vi "Read IP.vi"(8 "error in (no error)":errorcluster, 11 "RSeries_CAM in":refnum<class "RSeries_CAM.lvclass">) -> (0 "error out":errorcluster, 2 "IP":string, 3 "RSeries_CAM out":refnum<class "RSeries_CAM.lvclass">)   [LabVIEW 2024, in "RSeries_CAM.lvlib" / "RSeries_CAM.lvclass"]
uses:
  RSeries_CAM.lvclass
  RSeries_CAM.lvclass/RSeries_CAM.ctl
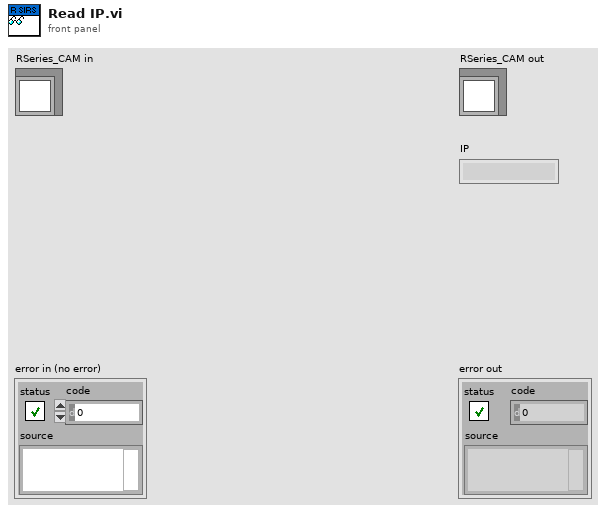
[diagram p1: front panel]
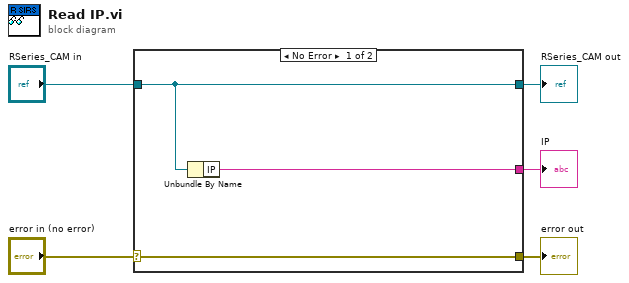
[diagram p0: block diagram]
diagram:
  n1 = case shown="No Error" "error in (no error)" {
    selector: "error in (no error)" -> [w8 w9]
    tunnel: [w8 w9] -> w4
    tunnel: [w7 w10] -> w2
    tunnel: "RSeries_CAM in" -> [w7 w10]
    tunnel: [w6 _] -> w1
    frame No Error {
      n2 = Unbundle By Name(w7) -> ("IP"=w6:string)
    }
    frame Error {
    }
  }
  "error out" <- w4
  "RSeries_CAM out" <- w2
  "IP" <- w1
